vi "ForLoop.vi"() -> ()   [LabVIEW 2023]
panel:
  out "Iterations":i32
  out "number (0 to 1)":dbl
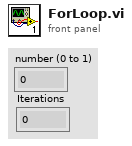
[diagram p1: front panel]
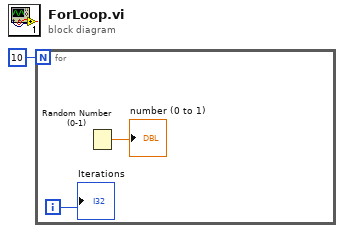
[diagram p0: block diagram]
diagram:
  n1 = for {
    N: 10 -> [_]
    i -> [w2]
    n2 = Random Number (0-1)() -> (number: 0 to 1=→"number (0 to 1)":dbl)
    "Iterations" <- w2
  }
